vi "soundGen.vi"(6 "Audio\nSafety":bool=TRUE caption="Audio", 8 "Trigger":bool, 9 "Audio\nDuration":dbl, 10 "Pattern \nFrequency":dbl, 11 "Frequency":dbl) -> ()   [LabVIEW 2010]
uses:
  <vilib>/measure/NI_MABase.lvlib
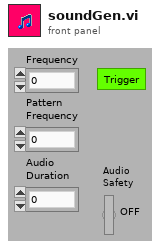
[diagram p1: front panel]
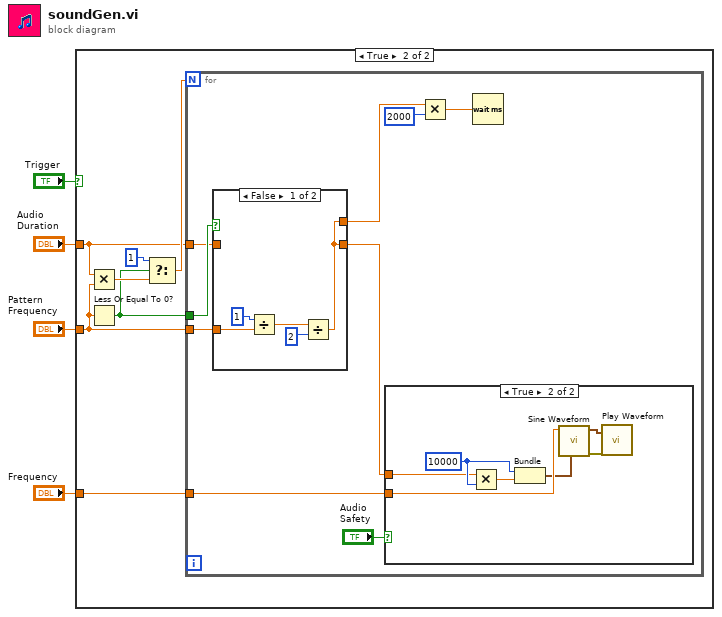
[diagram p0: block diagram]
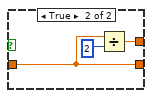
[diagram p4: hidden frame]
diagram:
  n1 = case shown="True" "Trigger" {
    tunnel: "Frequency" -> [_ w11]
    tunnel: "Audio\nDuration" -> [_ w6]
    tunnel: "Pattern \nFrequency" -> [_ w10]
    frame False {
    }
    frame True {
      n2 = Multiply(x=w6, y=w10) -> (x*y=w9:dbl)
      n3 = Less Or Equal To 0?(x=w10) -> (x <= 0?=w7:bool)
      n4 = Select(t=1, s=w7, f=w9) -> (s? t:f=w8:dbl)
      n5 = for {
        N: w8 -> [_]
        tunnel: w11 -> [w20]
        tunnel: w10 -> [w18]
        tunnel: w7 -> [w19]
        tunnel: w6 -> [w14]
        n6 = case shown="False" w19 {
          tunnel: w18 -> [w29 _]
          tunnel: [w28 w35] -> w13
          tunnel: [w28 w33] -> w15
          tunnel: w14 -> [_ w35]
          frame False {
            n7 = Divide(x=1, y=w29) -> (x/y=w30:dbl)
            n8 = Divide(x=w30, y=2) -> (x/y=w28:dbl)
          }
          frame True {
            n9 = Divide(x=w35, y=2) -> (x/y=w33:dbl)
          }
        }
        n10 = case shown="True" "Audio\nSafety" {
          tunnel: w20 -> [_ w27]
          tunnel: w13 -> [_ w21]
          frame False {
          }
          frame True {
            w26 = 10000
            n11 = Multiply(x=w21, y=w26) -> (x*y=w25:dbl)
            n12 = Bundle(w26, w25) -> (w24:cluster{i32, dbl})  [unwired: 1 in]
            n13 = call <vilib>:"Sine Waveform.vi"("sampling info"=w24, "frequency"=w27) -> ("error out"=w22:errorcluster, "signal out"=w23:waveform(dbl))  [unwired: 8 in]
            n14 = call "Play Waveform"("Data"=w23, "error in"=w22) -> ()  [unwired: 17 in, 1 out]
          }
        }
        n15 = Multiply(x=w15, y=2000) -> (x*y=w17:dbl)
        n16 = Wait (ms)(milliseconds to wait=w17) -> ()  [unwired: 1 out]
      }
    }
  }
